vi "02 LV - Real API list + loop.vi"() -> ()   [LabVIEW 2020]
uses:
  client/Client/Client.lvclass
  client/List/List.lvclass
  client/Asset/Asset.lvclass
panel:
  out "Found Items":string[](array[string])
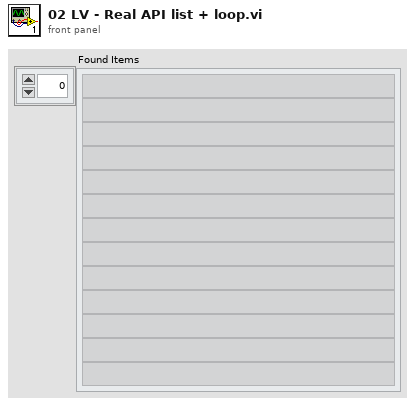
[diagram p1: front panel]
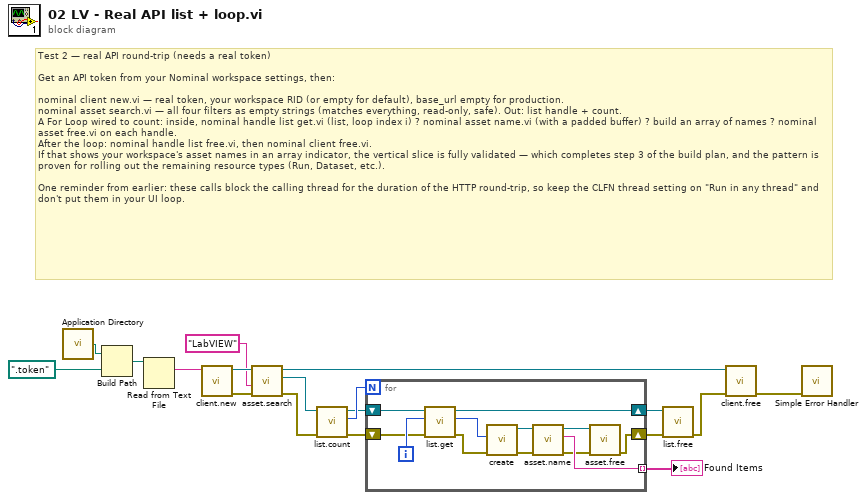
[diagram p0: block diagram]
diagram:
  # "Test 2 — real API round-trip (needs a real token)\n\nGet an API token from your Nominal workspace settings, then:\n\nnominal client new.vi — real token, your workspace RID (or empty for default), base_url empty for production.\nnominal asset search.vi — all four filters as empty strings (matches everything, read-only, safe). Out: list handle + count.\nA For Loop wired to count: inside, nominal handle list get.vi (list, loop index i) ? nominal asset name.vi (with a padded buffer) ? build an array of names ? nominal asset free.vi on each handle.\nAfter the loop: nominal handle list free.vi, then nominal client free.vi.\nIf that shows your workspace's asset names in an array indicator, the vertical slice is fully validated — which completes step 3 of the build plan, and the pattern is proven for rolling out the remaining resource types (Run, Dataset, etc.).\n\nOne reminder from earlier: these calls block the calling thread for the duration of the HTTP round-trip, so keep the CLFN thread setting on \"Run in any thread\" and don't put them in your UI loop."
  n1 = call <vilib>:"Application Directory.vi"() -> ("Application Directory"=w18:path)
  n2 = Build Path(base path=w18, name or relative path=path ".token") -> (appended path=w16:path)
  n3 = Read from Text File(file (use dialog)=w16) -> (text=w15:string)  [unwired: 3 in, 3 out]
  n4 = call "client.new.vi"("token"=w15) -> ("error out"=w13:errorcluster, "Client out"=w14:refnum<class "Client.lvclass">)  [unwired: 9 in]
  n5 = call "asset.search.vi"("error in"=w13, "label"="LabVIEW", "Client in"=w14) -> ("error out"=w1:errorcluster, "List"=w5:refnum<class "List.lvclass">, "Client out"=w8:refnum<class "Client.lvclass">)  [unwired: 6 in]
  n6 = call "list.count.vi"("error in"=w1, "List in"=w5) -> ("error out"=w2:errorcluster, "count"=w4:u32, "List out"=w3:refnum<class "List.lvclass">)  [unwired: 7 in]
  n7 = for {
    N: w4 -> [_]
    shift-right: [w19] -> w10
    shift-left: w2 -> [w28]
    shift-right: [w27] -> w11
    shift-left: w3 -> [w29]
    tunnel: [w21] -> w6 mode=indexing
    i -> [w30]
    n8 = call "list.get.vi"("error in"=w28, "index"=w30, "List in"=w29) -> ("error out"=w25:errorcluster, "handle"=w26:i32, "List out"=w27:refnum<class "List.lvclass">)  [unwired: 6 in]
    n9 = call "create.vi"("error in (no error)"=w25, "handle"=w26) -> ("error out"=w23:errorcluster, "Asset out"=w24:refnum<class "Asset.lvclass">)  [unwired: 8 in]
    n10 = call "asset.name.vi"("error in"=w23, "asset in"=w24) -> ("error out"=w20:errorcluster, "name"=w21:string, "asset out"=w22:refnum<class "Asset.lvclass">)  [unwired: 7 in]
    n11 = call "asset.free.vi"("error in"=w20, "asset in"=w22) -> ("error out"=w19:errorcluster)  [unwired: 9 in]
  }
  "Found Items" <- w6
  n12 = call "list.free.vi"("error in"=w10, "List in"=w11) -> ("error out"=w9:errorcluster)  [unwired: 9 in]
  n13 = call "client.free.vi"("error in"=w9, "Client in"=w8) -> ("error out"=w7:errorcluster)  [unwired: 9 in]
  n14 = call <vilib>:"Simple Error Handler.vi"("error in (no error)"=w7) -> ()  [unwired: 4 in, 5 out]
